vi "op_read.vi"(0 "Chain IN":bool) -> (4 "Chain OUT":bool, 6 "Encoder Left Drive":i32, 8 "Encoder Right Drive":i32, 10 "Moving Left Drive":bool, 15 "Moving Right Drive":bool)   [LabVIEW 2010, in "LASA Beta.lvrbt"]
uses:
  LASA Beta.lvrbt
  <vilib>/NXT/NXTIO Xnodes/AddressXNode/NXTIOAddress.xnode
  <vilib>/NXT/Subs/MotorXNode.DC Motor Type.ctl
  <vilib>/NXT/Subs/MotorXNode.2DCMotor.ctl
  <vilib>/NXT/Subs/LVHSConnector.ctl
  <vilib>/NXT/NXTIO Xnodes/NXTIOXNode/NXTIO.xnode
  <vilib>/NXT/NXTIO Xnodes/NXTIONodeSubVIs/TETRIX IO Motor Status.vi
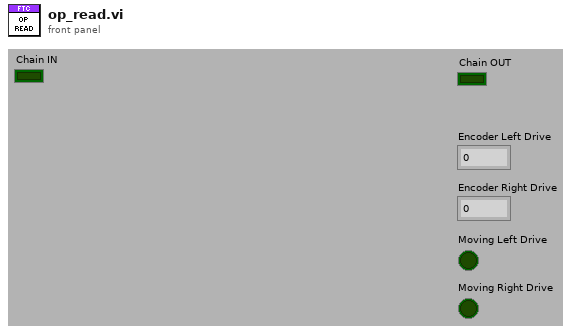
[diagram p1: front panel]
types:
  T1 = typedef "MotorXNode.DC Motor Type.ctl" = enum16{"DC Motor"}
  T2 = cluster{"DC Motor":T1, "Address":i16, "Address":i16}
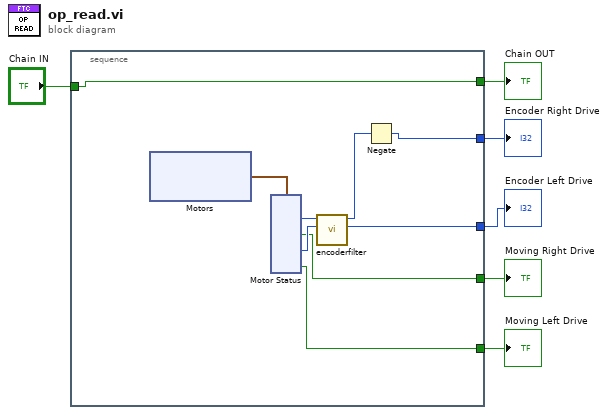
[diagram p0: block diagram]
diagram:
  n1 = stacked-sequence {
    tunnel: [w11] -> w6
    tunnel: [w10] -> w5
    tunnel: [w9] -> w4
    tunnel: [w8] -> w3
    tunnel: "Chain IN" -> [w7]
    tunnel: [w7] -> w1
    frame #0 {
      n2 = xnode "Motors"() -> ("DC Motor"=w15:T2)
      n3 = xnode "Motor Status"("Motors"=w15) -> ("Moving 2"=w8:bool, "Moving 1"=w9:bool, "Position 2"=w13:i32, "Position 1"=w14:i32)  [unwired: 1 in, 1 out]
      n4 = call "encoderfilter.vi"("Encoder Input 2"=w13, "Encoder Input"=w14) -> ("Encoder Output 2"=w10:i32, "Encoder Output"=w12:i32)  [unwired: 6 in, 2 out]
      n5 = Negate(x=w12) -> (-x=w11:i32)
    }
  }
  "Encoder Left Drive" <- w5
  "Encoder Right Drive" <- w6
  "Moving Left Drive" <- w3
  "Moving Right Drive" <- w4
  "Chain OUT" <- w1
